vi "Create connection (SubVI).vi"(2 "error in (no error)":errorcluster, 3 "host name":string, 4 "Connection in":refnum<class "Connection.lvclass">) -> (0 "error out":errorcluster, 1 "Connection out":refnum<class "Connection.lvclass">)   [LabVIEW 2016]
doc: "Create a connection using the username and password in the amqp info global variable."
uses:
  <vilib>/Distrio/LabbitMQ/Connection/Connection.lvclass
  <vilib>/Distrio/LabbitMQ/Connection/connection_parameters_cluster.ctl
  global/AMQP_credentials.vi
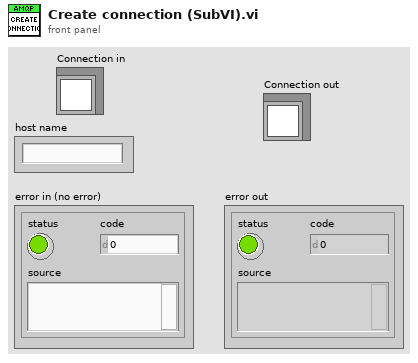
[diagram p1: front panel]
types:
  T1 = typedef "Connection.lvclass/connection_parameters_cluster.ctl" = cluster{"host name":string, "port":i32, "user name":string, "password":string, "virtual host":string}
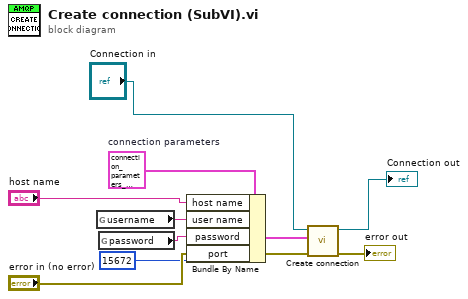
[diagram p0: block diagram]
diagram:
  w9 = T1 {"host name"="localhost", "port"=5672, "user name"="guest", "password"="guest", "virtual host"="/"}  # connection parameters
  n1 = global read "AMQP_credentials.vi" "username"() -> (w7:string)
  n2 = global read "AMQP_credentials.vi" "password"() -> (w6:string)
  n3 = Bundle By Name(cluster=w9, "host name"="host name", "user name"=w7, "password"=w6, "port"=15672) -> (w8:T1)
  n4 = call <vilib>:"Create connection.vi"("error in (no error)"="error in (no error)", "connection parameters"=w8, "Connection in"="Connection in") -> ("error out"=→"error out":errorcluster, "Connection out"=→"Connection out":refnum<class "Connection.lvclass">)  [unwired: 7 in]
